vi "niRFUtil LCAPI Copy 1D Array (3 DBL).vi"(0 "Source0 1D Array (DBL)":dbl[](array[numeric]) format="%.2f", 5 "Source1 1D Array (DBL)":dbl[](array[numeric]) format="%.2f", 7 "Source2 1D Array (DBL)":dbl[](array[numeric]) format="%.2f", 11 "error in (no error)":errorcluster, 12 "Data Copy Descriptor":u64) -> (4 "Source0 Out":dbl[](array[numeric]) format="%.2f", 6 "Source1 Out":dbl[](array[numeric]) format="%.2f", 8 "Source2 Out":dbl[](array[numeric]) format="%.2f", 15 "error out":errorcluster)   [LabVIEW 2015, in "niRFUtil.lvlib"]
uses:
  niRFUtil.lvlib
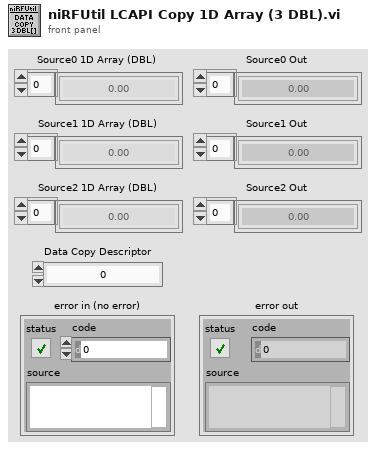
[diagram p1: front panel]
types:
  T1 = cluster{"status":bool, "return type":i32, "errorString":string}
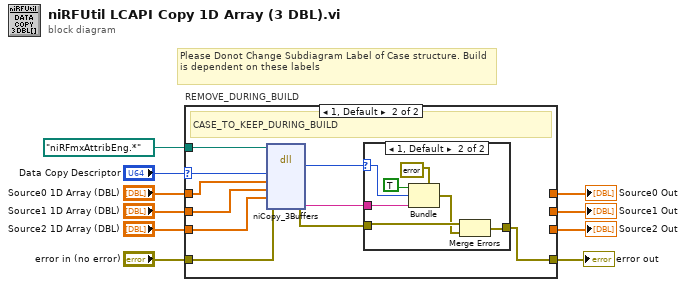
[diagram p0: block diagram]
diagram:
  # "Please Donot Change Subdiagram Label of Case structure. Build is dependent on these labels"
  n1 = case "REMOVE_DURING_BUILD" shown="1, Default" "Data Copy Descriptor" {
    selector: "Data Copy Descriptor" -> [_ w16]
    tunnel: "error in (no error)" -> [w14 w23]
    tunnel: "Source0 1D Array (DBL)" -> [w11 w22]
    tunnel: "Source1 1D Array (DBL)" -> [w12 w21]
    tunnel: "Source2 1D Array (DBL)" -> [w13 w20]
    tunnel: [w14 w24] -> w5
    tunnel: [w13 _] -> w4
    tunnel: [w12 _] -> w3
    tunnel: [w11 _] -> w2
    tunnel: path "niRFmxAttribEng.*" ("path in") -> [_ w15]
    frame 0 {
      # "Development"
    }
    frame 1, Default {
      # "CASE_TO_KEEP_DURING_BUILD"
      n2 = dll-call lib="niRFmxAttribEng.*" fn="niCopy_3Buffers"(path in=w15, error in=w23, "dataCopyDescriptor"=w16, "source0"=w22, "source1"=w21, "source2"=w20) -> (error out=w18:errorcluster, "return type"=w19:i32, "errorString"=w17:string)  [unwired: 6 in, 1 out]
      n3 = case shown="1, Default" w19 {
        selector: w19 -> [_ w31]
        tunnel: w17 -> [_ w30]
        tunnel: w18 -> [w25 w28]
        tunnel: [w25 w29] -> w24
        frame 0 {
        }
        frame 1, Default {
          n4 = Bundle(cluster=T1 {"status"=FALSE, "return type"=0, "errorString"=""}, "status"=TRUE, "return type"=w31, "errorString"=w30) -> (w27:T1)
          n5 = Merge Errors(w28, w27) -> (w29:errorcluster)
        }
      }
    }
  }
  "error out" <- w5
  "Source0 Out" <- w2
  "Source1 Out" <- w3
  "Source2 Out" <- w4
